vi "释放内存.vi"   [LabVIEW 2014]
uses:
  FreeMem.dll
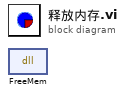
[diagram p0: block diagram]
diagram:
  n1 = dll-call lib="C:/Users/p-c/Desktop/FreeMem/FreeMem.dll" fn="FreeMem"() -> ()  [unwired: 4 in, 2 out]
